vi "Basic_20230215.vi"() -> ()   [LabVIEW 2021, in "GettingStarted_5774_Host.lvlib"]
uses:
  GettingStarted_5774_Host.lvlib
  <vilib>/userDefined/High Color/nirio_resource_hc.ctl
  <instrlib>/FlexRIO/API/Host/v1/NI FlexRIO/API/Reference Clock Source.ctl
  <instrlib>/FlexRIO/API/Host/v1/NI FlexRIO/API/Get Property Reference - Fpga Small.vi
  <instrlib>/FlexRIO/API/Host/v1/NI FlexRIO/API/Configure Analog Start Trigger.vi
  <instrlib>/FlexRIO/API/Host/v1/NI FlexRIO/API/Configure Digital Edge Start Trigger.vi
  <instrlib>/FlexRIO/API/Host/v1/NI FlexRIO/API/Configure Immediate Start Trigger.vi
  <instrlib>/FlexRIO/API/Host/v1/NI FlexRIO/API/Read Stream 1D WDT.vi
  <vilib>/measure/maspectr.llb/FFT Power Spectrum and PSD for N Chan.vi
  <vilib>/FPGAPlugInAG/Dynamic/niLvFpga_Close_Dynamic.vi
  <vilib>/rvi/interface/nirviCloseFPGA/nirviCloseFPGA.xnode
  <instrlib>/FlexRIO/API/Host/v1/NI FlexRIO/API/Configure Reference Clock.vi
  <instrlib>/FlexRIO/API/Host/v1/NI FlexRIO API v1.lvlib
  <resource>/objmgr/niflexrioapiStream.rc
  <vilib>/measure/NI_MAPro.lvlib
  <resource>/objmgr/niflexrioapiChannel.rc
panel:
  in  "reference clock source":T1 items=["Default", "Onboard", "PXI_Clk10", "External", "None", "Baseboard Reference"]
  in  "AI1 Range":dbl(ring)=1.0 items=["1V"=1.0, "200mV"=0.2]
  in  "AI0 Range":dbl(ring)=1.0 items=["1V"=1.0, "200mV"=0.2]
  in  "AI1 Offset (V)":dbl
  in  "AI0 Offset (V)":dbl
  out "Sample Rate":dbl=3200000000.0 format="%#_6p"
  in  "ADC Interleaving Factor":i32=1 min=0 max=2 step=1
  in  "AI num samples":u64=320 step=16
  in  "AI channels":string="AI0,AI1"
  out "Device Power":dbl(slide) scale=-1.0..38.0 scale format="%#_3p"
  out "FPGA Temperature":dbl(slide) scale=0.0..100.0 scale format="%#_3p"
  in  "Trigger Type":enum32{"Immediate", "Analog", "Digital"}(tab)
  in  "trigger channel":string(combo)="AI0"
  in  "rising edge?":bool=TRUE
  in  "level (V)":dbl format="%#_3p"
  in  "hysteresis (V)":dbl format="%#_3p"
  in  "digital trigger source":string(combo)
  in  "stop":bool
  in  "Waveform Tab Control":enum32{"AI Time Domain", "AI Frequency Domain"}(tab)
  out "Waveform Graph":waveform(dbl)[](graph)
  out "FFT":cluster{"f0":dbl, "df":dbl, "magnitude":dbl[]}[](graph) caption="Waveform Graph"
  out "error out":errorcluster
  out "Limit (W)":dbl
  out "Power (W)":dbl
  out "Limit (C)":dbl
  out "Temp (C)":dbl format="%#_4p"
  in  "RIO Device":T2
  # "Overview: Configure an acquisition for a FlexRIO target and transfer the data to the host using the FlexRIO Host API.  Loop an output waveform\nRequirements: FlexRIO\nInstructions: \n 1. Select the RIO Device that corresponds to the FlexRIO target. \n 2. Optionally configure the clocking, stream, and trigger. \n 3. Run the VI"
  # "Resource Configuration"
  # "Clocking configuration"
  # "Input Waveform Configuration"
  # "Device Monitoring"
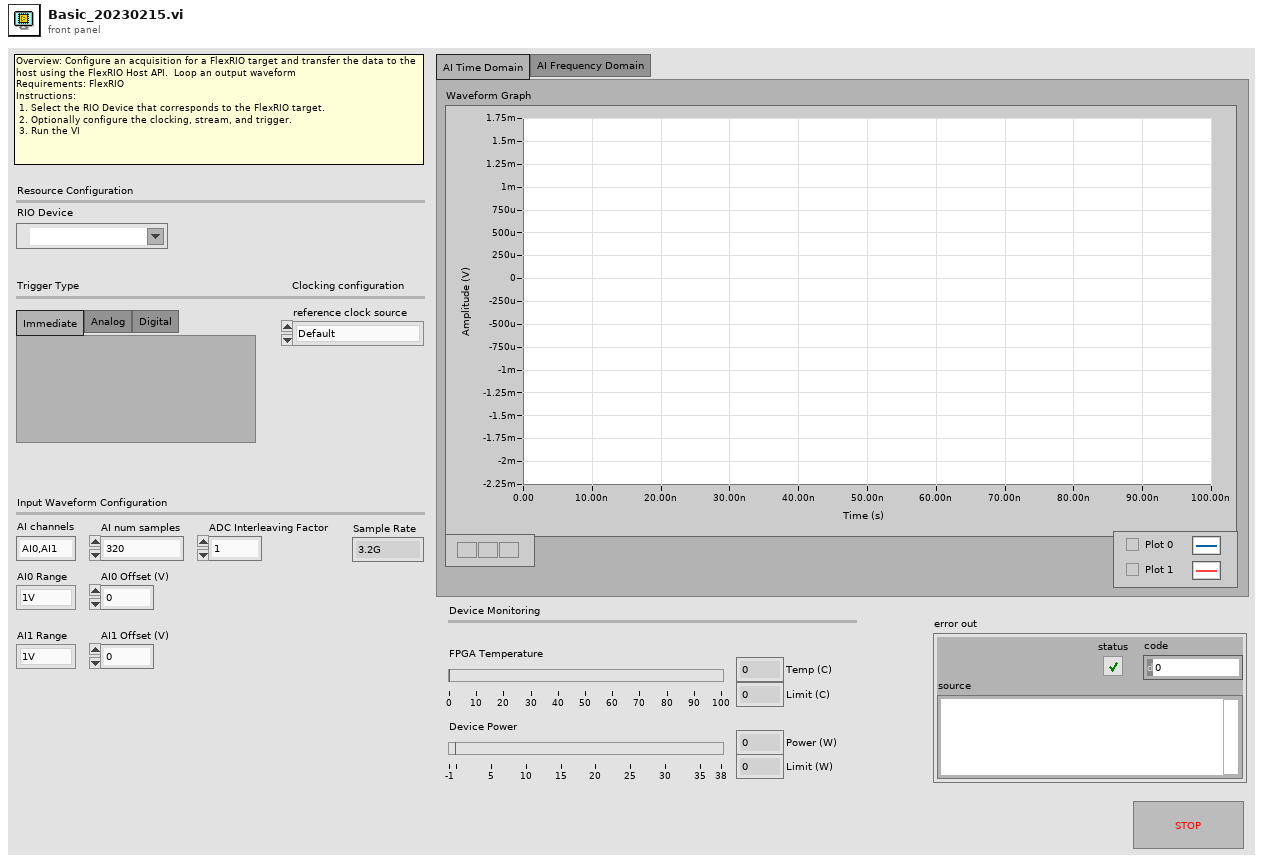
[diagram p1: front panel]
types:
  T1 = typedef "NI FlexRIO API v1.lvlib/Reference Clock Source.ctl" = i32
  T2 = typedef "nirio_resource_hc.ctl" = tag
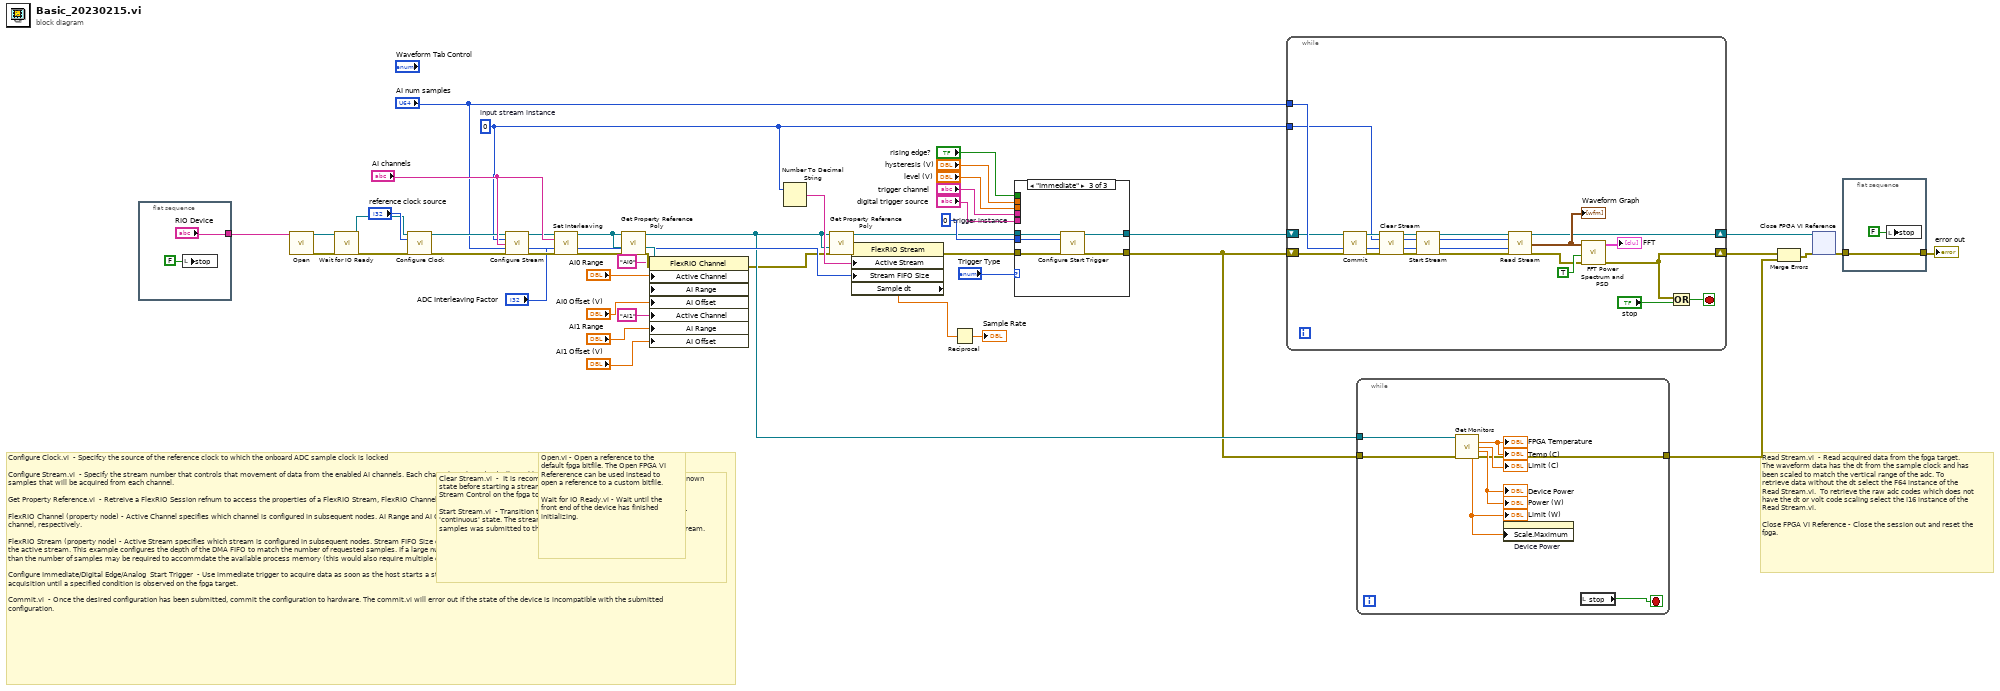
[diagram p0: block diagram]
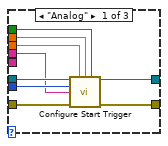
[diagram p2: hidden frame]
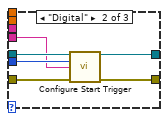
[diagram p3: hidden frame]
diagram:
  w12 = u32 0  # trigger instance
  w10 = u32 0  # input stream instance
  # "Read Stream.vi  - Read acquired data from the fpga target. The waveform data has the dt from the sample clock and has been scaled to match the vertical range of the adc. To retrieve data without the dt select the F64 instance of the Read Stream.vi.  To retrieve the raw adc codes which does not have the dt or volt code scaling select the I16 instance of the Read Stream.vi.  \n\nClose FPGA VI Reference - Close the session out and reset the fpga."
  # "Clear Stream.vi  -  It is recommended practice to put the stream into a known state before starting a stream. Calling Clear Stream.vi  commands the Stream Control on the fpga to transition to the 'idle' state.\n\nStart Stream.vi  - Transition the stream from an 'idle' state to a 'finite' or 'continuous' state. The stream will transition to 'finite' if a non zero num samples was submitted to the configure stream.vi before starting the stream."
  # "Configure Clock.vi  - Specifcy the source of the reference clock to which the onboard ADC sample clock is locked\n\nConfigure Stream.vi  - Specify the stream number that controls that movement of data from the enabled AI channels. Each channel can be individually enabled or disabled. Specify the number of samples that will be acquired from each channel. \n\nGet Property Reference.vi  - Retreive a FlexRIO Session refnum to access the properties of a FlexRIO Stream, FlexRIO Channel, FlexRIO Trigger, or FlexRIO Properties.\n\nFlexRIO Channel (property node) - Active Channel specifies which channel is configured in subsequent nodes. AI Range and AI Offset configure the vertical input range and offset for the specified channel, respectively.\n\nFlexRIO Stream (property node) - Active Stream specifies which stream is configured in subsequent nodes. Stream FIFO Size configures the depth of the host side DMA FIFO for the channels owned by the active stream. This example configures the depth of the DMA FIFO to match the number of requested samples. If a large number of samples is requested in LabVIEW 32 bit, a FIFO depth smaller than the number of samples may be required to accommdate the available process memory (this would also require multiple calls to the Read Stream.vi to retrieve all acquired but unfetched data). \n\nConfigure Immediate/Digital Edge/Analog  Start Trigger  - Use immediate trigger to acquire data as soon as the host starts a stream. Digital or analog trigger modes will defer the start of an acquisition until a specified condition is observed on the fpga target. \n\nCommit.vi  - Once the desired configuration has been submitted, commit the configuration to hardware. The commit.vi will error out if the state of the device is incompatible with the submitted configuration."
  # "Open.vi - Open a reference to the default fpga bitfile. The Open FPGA VI Refererence can be used instead to open a reference to a custom bitfile.\n\nWait for IO Ready.vi - Wait until the front end of the device has finished initializing."
  n1 = flat-sequence {
    tunnel: ["RIO Device"] -> w1
    frame #0 {
      n2 = local write "stop"(FALSE ("stop")) -> ()
    }
  }
  n3 = call <instrlib>:"Open.vi"("RIO Device"=w1) -> ("fpga interface out"=w45:refnum<k20>, "error out"=w46:errorcluster)  [unwired: 13 in]
  n4 = call <instrlib>:"Wait for IO Ready.vi"("fpga interface in"=w45, "error in"=w46) -> ("fpga interface out"=w16:refnum<k20>, "error out"=w15:errorcluster)  [unwired: 10 in, 2 out]
  n5 = call-poly <instrlib>:"Configure Clock.vi"("fpga interface in"=w16, "reference clock source"="reference clock source", "error in"=w15) -> ("fpga interface out"=w21:refnum<k20>, "error out"=w22:errorcluster)  [unwired: 11 in]
  n6 = call <instrlib>:"Configure Stream.vi"("fpga interface in"=w21, "stream instance"=w10, "channels enabled"="AI channels", "num samples"="AI num samples", "error in"=w22) -> ("fpga interface out"=w29:refnum<k20>, "error out"=w30:errorcluster)  [unwired: 7 in, 2 out]
  n7 = call "Set Interleaving.vi"("fpga interface in"=w29, "AI channels enabled"="AI channels", "ADC Interleaving Factor"="ADC Interleaving Factor", "error in (no error)"=w30) -> ("fpga interface out"=w8:refnum<k20>, "error out"=w39:errorcluster)  [unwired: 10 in]
  n8 = call-poly <instrlib>:"Get Property Reference Poly.vi"("error in (no error)"=w39, "fpga interface in"=w8) -> ("error out"=w38:errorcluster, "property reference"=w37:refnum<k20>)  [unwired: 4 in, 1 out]
  n9 = property class="FlexRIO Channel"(reference=w37, error in=w38, "Active Channel"="AI0" ("Active Stream"), "AI Range"="AI0 Range", "AI Offset"="AI0 Offset (V)", "Active Channel"="AI1" ("Active Stream"), "AI Range"="AI1 Range", "AI Offset"="AI1 Offset (V)") -> (error out=w6:errorcluster)  [unwired: 1 out]
  n10 = Number To Decimal String(number=w10) -> (decimal integer string=w23:string)  [unwired: 1 in]
  n11 = call-poly <instrlib>:"Get Property Reference Poly.vi"("error in (no error)"=w6, "fpga interface in"=w8) -> ("error out"=w31:errorcluster, "property reference"=w32:refnum<k20>)  [unwired: 4 in, 1 out]
  n12 = property class="FlexRIO Stream"(reference=w32, error in=w31, "Active Stream"=w23, "Stream FIFO Size"="AI num samples") -> (error out=w26:errorcluster, "Sample dt"=w27:dbl)  [unwired: 1 out]
  n13 = Reciprocal(x=w27) -> (1/x=→"Sample Rate":dbl)
  n14 = case shown="\"Immediate\"" "Trigger Type" {
    tunnel: w8 -> [w57 w63 w68]
    tunnel: w26 -> [w56 w62 w67]
    tunnel: [w55 w61 w66] -> w9
    tunnel: [w54 w60 w65] -> w7
    tunnel: w12 -> [w53 w59 w64]
    tunnel: "trigger channel" -> [w52 _ _]
    tunnel: "level (V)" -> [w51 _ _]
    tunnel: "hysteresis (V)" -> [w50 _ _]
    tunnel: "rising edge?" -> [w49 _ _]
    tunnel: "digital trigger source" -> [_ w58 _]
    frame "Analog" {
      n15 = call-poly <instrlib>:"Configure Start Trigger.vi"("fpga interface in"=w57, "level"=w51, "hysteresis"=w50, "rising edge?"=w49, "trigger instance"=w53, "channel"=w52, "error in"=w56) -> ("fpga interface out"=w55:refnum<k20>, "error out"=w54:errorcluster)  [unwired: 6 in, 1 out]
    }
    frame "Digital" {
      n16 = call-poly <instrlib>:"Configure Start Trigger.vi"("fpga interface in"=w63, "trigger instance"=w59, "trigger source"=w58, "error in"=w62) -> ("fpga interface out"=w61:refnum<k20>, "error out"=w60:errorcluster)  [unwired: 9 in, 1 out]
    }
    frame "Immediate" {
      n17 = call-poly <instrlib>:"Configure Start Trigger.vi"("fpga interface in"=w68, "trigger instance"=w64, "error in"=w67) -> ("fpga interface out"=w66:refnum<k20>, "error out"=w65:errorcluster)  [unwired: 10 in, 1 out]
    }
  }
  n18 = while {
    shift-right: [w81] -> w43
    shift-left: w7 -> [w70]
    shift-right: [w85] -> w44
    shift-left: w9 -> [w72]
    tunnel: "AI num samples" -> [w80]
    tunnel: w10 -> [w74]
    stop <- w83 stop-if-true
    n19 = call <instrlib>:"Commit.vi"("fpga interface in"=w72, "error in"=w70) -> ("fpga interface out"=w75:refnum<k20>, "error out"=w76:errorcluster)  [unwired: 12 in]
    n20 = call <instrlib>:"Clear Stream.vi"("fpga interface in"=w75, "stream instance"=w74, "error in"=w76) -> ("fpga interface out"=w79:refnum<k20>, "stream instance out"=w78:u32, "error out"=w77:errorcluster)  [unwired: 10 in]
    n21 = call <instrlib>:"Start Stream.vi"("fpga interface in"=w79, "stream instance"=w78, "error in"=w77) -> ("fpga interface out"=w71:refnum<k20>, "stream instance out"=w73:u32, "error out"=w69:errorcluster)  [unwired: 10 in]
    n22 = call-poly <instrlib>:"Read Stream.vi"("fpga interface in"=w71, "stream instance"=w73, "samples"=w80, "error in"=w69) -> ("fpga interface out"=w85:refnum<k20>, "read data"=w87:waveform(dbl)[], "error out"=w82:errorcluster)  [unwired: 7 in, 2 out]
    "Waveform Graph" <- w87
    n23 = call-poly <vilib>:"FFT Power Spectrum and PSD.vi"("error in (no error)"=w82, "dB On (F)"=TRUE, "time signals"=w87) -> ("error out"=w81:errorcluster, "Power Spectrum / PSD"=→"FFT":cluster{"f0":dbl, "df":dbl, "magnitude":dbl[]}[])  [unwired: 5 in, 2 out]
    n24 = Or(x=w81, y="stop") -> (x .or. y?=w83:bool)
  }
  n25 = while {
    tunnel: w8 -> [w92]
    tunnel: w7 -> [w91]
    tunnel: [w89] -> w4
    stop <- w90 stop-if-true
    n26 = call "Get Monitors.vi"("fpga interface in"=w92, "error in (no error)"=w91) -> ("FPGA Temperature (C)"=→"Temp (C)" →"FPGA Temperature":dbl, "Temperature Limit (C)"=→"Limit (C)":dbl, "Total Power (W)"=→"Power (W)" →"Device Power":dbl, "Power Limit (W)"=w95:dbl, "error out"=w89:errorcluster)  [unwired: 8 in, 1 out]
    "Limit (W)" <- w95
    n27 = property on="Device Power" class="Slide (strict)"("Scale.Maximum"=w95) -> ()  [unwired: 2 in, 2 out]
    n28 = local read "stop"() -> (w90:bool)
  }
  n29 = Merge Errors(w43, w4) -> (w5:errorcluster)
  n30 = xnode "Close FPGA VI Reference"("FPGA VI Reference In"=w44, "error in"=w5) -> ("error out"=w3:errorcluster)
  n31 = flat-sequence {
    tunnel: w3 -> [w97]
    tunnel: [w97] -> w2
    frame #0 {
      n32 = local write "stop"(FALSE ("stop")) -> ()
    }
  }
  "error out" <- w2
